vi "GetEvtSignal.vi"(8 "error in (no error)":errorcluster, 11 "C37EventPlugin in":refnum<class "C37EvtPlugin.lvclass">) -> (0 "error out":errorcluster, 3 "C37EventPlugin out":refnum<class "C37EvtPlugin.lvclass">)   [LabVIEW 2014, in "EventPlugins.lvlib" / "C37EvtPlugin.lvclass"]
uses:
  C37EvtPlugin.lvclass
  EventPluginBaseClass/Accessors/Read EvtConfig.vi
  EventPluginBaseClass/Accessors/Read TimeArray.vi
  EventPluginBaseClass/Accessors/Read EvtParams.vi
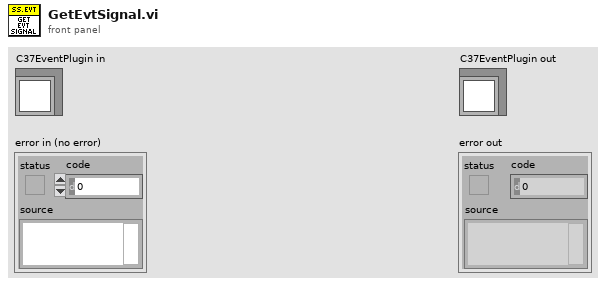
[diagram p1: front panel]
types:
  T1 = typedef "EventPlugins.lvlib/EventPluginBaseClass.lvclass/clEvtConfig.ctl" = cluster{"T0(UTC)":dbl, "F0":dbl, "Fs":i32, "FSamp":u32, "bPosSeq":bool}
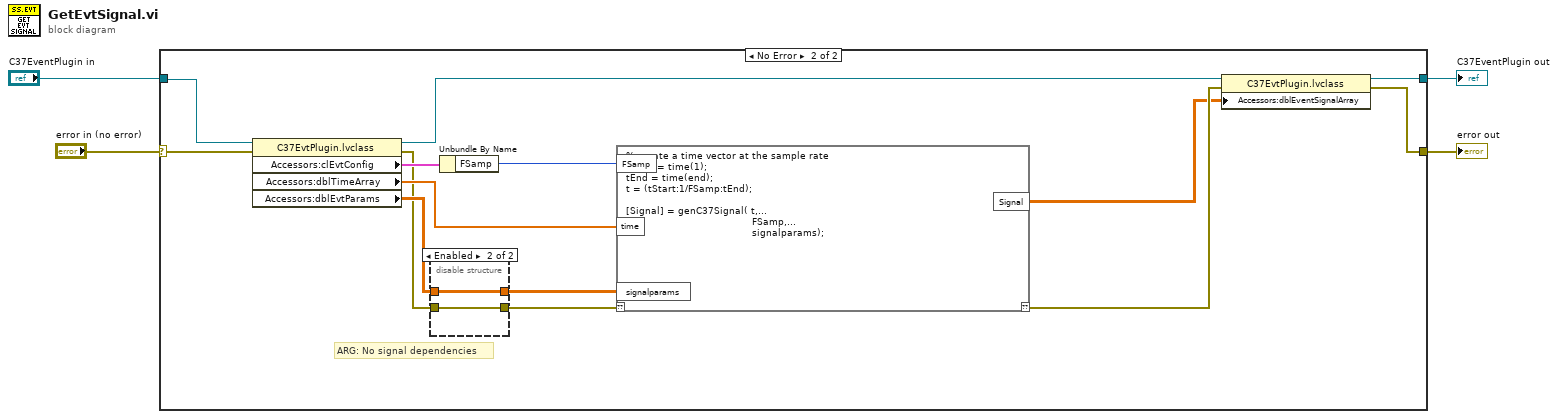
[diagram p0: block diagram]
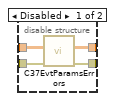
[diagram p3: hidden frame]
diagram:
  n1 = case shown="No Error" "error in (no error)" {
    selector: "error in (no error)" -> [w6 w17]
    tunnel: [w5 w20] -> w4
    tunnel: "C37EventPlugin in" -> [w5 w18]
    tunnel: [w6 w19] -> w3
    frame Error {
    }
    frame No Error {
      # "ARG: No signal dependencies"
      n2 = property class="C37EvtPlugin.lvclass"(reference=w18, error in=w17) -> (reference out=w14:refnum<class "C37EvtPlugin.lvclass">, error out=w8:errorcluster, "Accessors:clEvtConfig"=w16:T1, "Accessors:dblTimeArray"=w12:dbl[], "Accessors:dblEvtParams"=w9:dbl[][])
      n3 = disable-structure shown="Enabled" {
        disable-tunnel: [w24 w25] -> w11
        disable-tunnel: [w23 w26] -> w10
        disable-tunnel: w9 -> [w22 w26]
        disable-tunnel: w8 -> [w21 w25]
        frame Disabled {
          n4 = call "C37EvtParamsErrors.vi"("error in (no error)"=w21, "dblSignalParams in"=w22) -> ("error out"=w24:errorcluster, "dblSignalParams out"=w23:dbl[][])  [unwired: 8 in]
        }
        frame Enabled {
        }
      }
      n5 = Unbundle By Name(w16) -> ("FSamp"=w15:u32)
      n6 = script code="% create a time vector at the sample rate\ntStart = time(1);\ntEnd = time(end);\nt = (tStart:1/FSamp:tEnd);\n\n[Signal] = genC37Signal( t,...\n                                          FSamp,...\n                                          signalparams);"("??"=w11, "FSamp"=w15, "time"=w12, "signalparams"=w10) -> ("??"=w13:errorcluster, "Signal"=w7:dbl[][])
      n7 = property class="C37EvtPlugin.lvclass"(reference=w14, error in=w13, "Accessors:dblEventSignalArray"=w7) -> (reference out=w20:refnum<class "C37EvtPlugin.lvclass">, error out=w19:errorcluster)
    }
  }
  "error out" <- w3
  "C37EventPlugin out" <- w4
